vi "Global - FileSync.vi"() -> ()   [LabVIEW 2020, in "FileSync -- Base.lvlib"]
uses:
  FileSync -- Base.lvlib
  Def-FileSyncConfig.ctl
panel:
  in  "FileSync Configuration":T1
  in  "Connected":bool
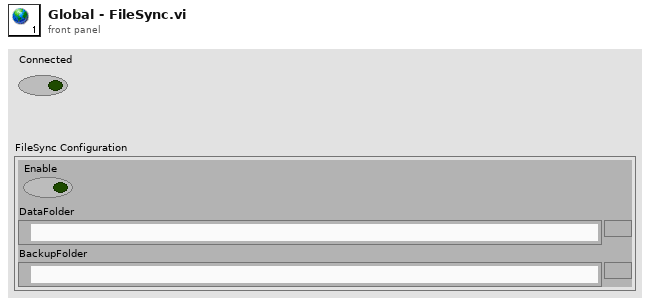
[diagram p1: front panel]
types:
  T1 = typedef "FileSync -- Base.lvlib/Def-FileSyncConfig.ctl" = cluster{"Enable":bool, "DataFolder":path, "BackupFolder":path}
diagram:
